vi "findTitles.vi"(7 "all rows in":string[][](array[string]), 10 "Array - String":string[](array[string])) -> (2 "titleColumn":i32, 5 "data":string[][](array[string]))   [LabVIEW 2020]
panel:
  # "Warning- no error checking for not found!"
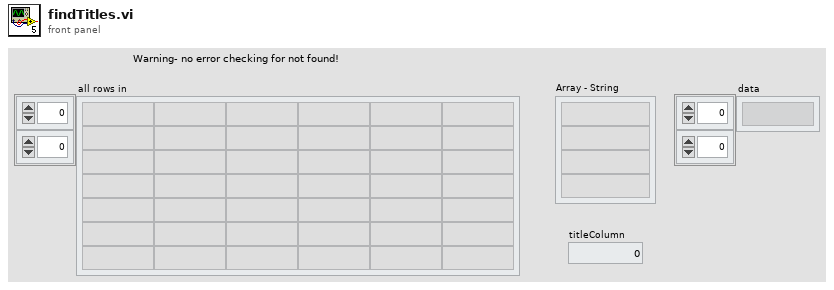
[diagram p1: front panel]
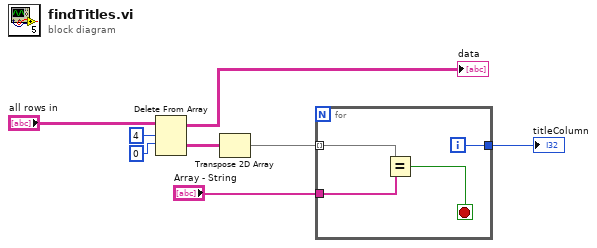
[diagram p0: block diagram]
diagram:
  n1 = Delete From Array(array="all rows in", length=4 ("index (row)"), index (row)=0 ("disabled index (col)")) -> (deleted portion=w2:string[][], array with subset deleted=→"data":string[][])  [unwired: 1 in]
  n2 = Transpose 2D Array(2D array=w2) -> (transposed array=w5:string[][])
  n3 = for {
    tunnel: w5 -> [w12] mode=indexing
    tunnel: "Array - String" -> [w11]
    tunnel: [w9] -> w3
    i -> [w9]
    stop <- w10 stop-if-true
    n4 = Equal?(x=w12, y=w11) -> (x = y?=w10:bool)
  }
  "titleColumn" <- w3
